vi "Add Logger to Map.vi"(8 "error in (no error)":errorcluster, 9 "Logger":refnum<class "Logger.lvclass">, 10 "Name":string, 11 "Registry in":refnum<class "Registry.lvclass">) -> (0 "error out":errorcluster, 3 "Registry out":refnum<class "Registry.lvclass">)   [LabVIEW 2020, in "LV Logging.lvlib" / "Registry.lvclass"]
uses:
  Registry.lvclass
  Logger/Logger.lvclass
  Registry.lvclass/Registry.ctl
  <vilib>/Utility/miscctls.llb/LVMapReplaceAction.ctl
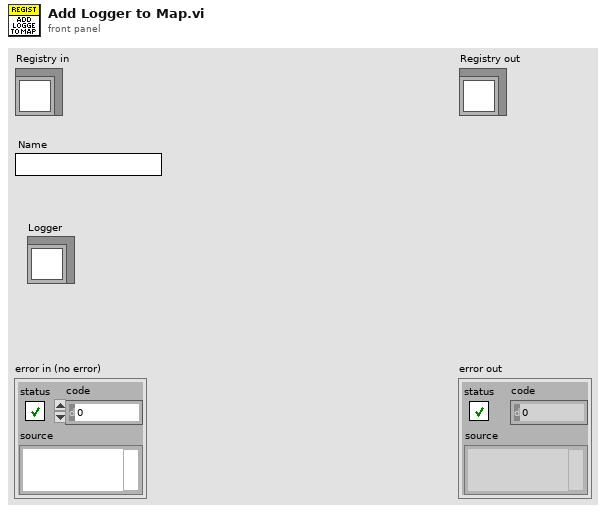
[diagram p1: front panel]
types:
  T1 = typedef "LVMapReplaceAction.ctl" = enum32{"Modify Entry only if found", "Add or Modify Entry", "Delete Entry"}
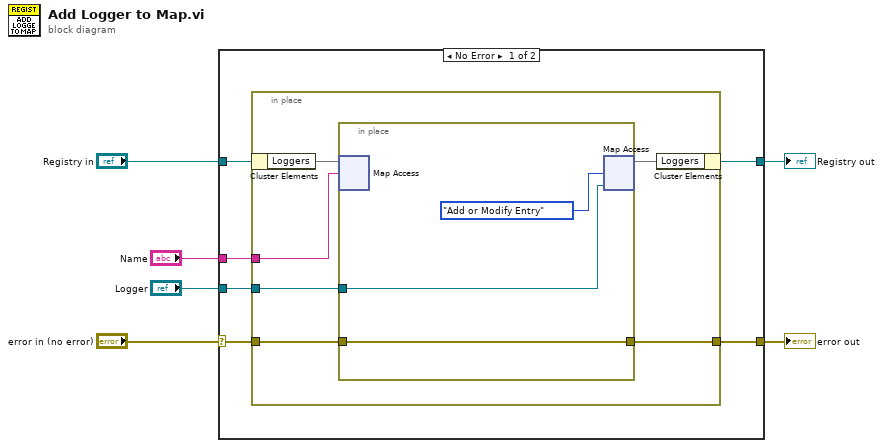
[diagram p0: block diagram]
diagram:
  n1 = case shown="No Error" "error in (no error)" {
    selector: "error in (no error)" -> [w11 w23]
    tunnel: [w12 w23] -> w5
    tunnel: [w9 w22] -> w3
    tunnel: "Registry in" -> [w10 w22]
    tunnel: "Name" -> [w8 _]
    tunnel: "Logger" -> [w7 _]
    frame No Error {
      n2 = in-place {
        in-place-border: [w18] -> w12
        in-place-border: w11 -> [w17]
        in-place-border: w8 -> [w14]
        in-place-border: w7 -> [w13]
        n3 = in-place-cluster #1(w10) -> ("Loggers"=w16:map{string, refnum<class "Logger.lvclass">})
        n4 = in-place {
          in-place-border: [w21] -> w18
          in-place-border: w17 -> [w21]
          in-place-border: w13 -> [w19]
          n5 = in-place-map #2(w16, w14) -> ()  [unwired: 1 in, 2 out]
          n6 = in-place-map #2(w19, LVMapReplaceAction."Add or Modify Entry" ("action")) -> (w15:map{string, refnum<class "Logger.lvclass">})  [unwired: 2 out]
        }
        n7 = in-place-cluster #1("Loggers"=w15) -> (w9:refnum<class "Registry.lvclass">)
      }
    }
    frame Error {
    }
  }
  "error out" <- w5
  "Registry out" <- w3
